vi "Get Disable.vi"(8 "error in (no error)":errorcluster, 11 "S4ACS_GUI in":refnum<class "S4GUI.lvclass">) -> (0 "error out":errorcluster, 3 "S4ACS_GUI out":refnum<class "S4GUI.lvclass">)   [LabVIEW 2018, in "S4GUI.lvclass"]
uses:
  S4GUI.lvclass
  S4GUI.lvclass/S4GUI.ctl
  Server/Server.lvclass/Server.ctl
  Acquisition/Acquisition.lvclass
  C:/Users/devstaff/sparc4/s4gui/Versao ZeroMQ REQ-REP/SPARC4_GUI -v1.0.9 - novo comportamento aba TEST/Server/Server.lvclass
  Instrument/Instrument.lvclass
  Server/Server.lvclass
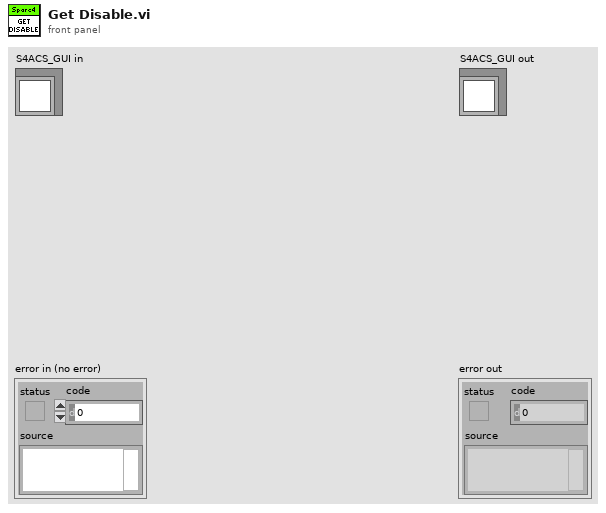
[diagram p1: front panel]
types:
  T1 = enum8{"Enabled", "Disabled", "Disabled and Grayed Out"}
  T2 = cluster{"Cluster Mode Sync":cluster{"#Index Cycles":enum8{"Enabled", "Disabled", "Disabled and Grayed Out"}, "#Cycles":enum8{"Enabled", "Disabled", "Disabled and Grayed Out"}, "SSM":enum8{"Enabled", "Disabled", "Disabled and Grayed Out"}, "Set SM":enum8{"Enabled", "Disabled", "Disabled and Grayed Out"}, "Star SM":enum8{"Enabled", "Disabled", "Disabled and Grayed Out"}, "Pause SM":enum8{"Enabled", "Disabled", "Disabled and Grayed Out"}, "Stop SM":enum8{"Enabled", "Disabled", "Disabled and Grayed Out"}, "Abort SM":enum8{"Enabled", "Disabled", "Disabled and Grayed Out"}, "Start SM Text":string}, "Cluster Polarimetry":cluster{"Lambda Selector":enum8{"Enabled", "Disabled", "Disabled and Grayed Out"}, "Calibrator Selector":enum8{"Enabled", "Disabled", "Disabled and Grayed Out"}, "Set Waveplate":enum8{"Enabled", "Disabled", "Disabled and Grayed Out"}, "Select Positions":enum8{"Enabled", "Disabled", "Disabled and Grayed Out"}, "P0":enum8{"Enabled", "Disabled", "Disabled and Grayed Out"}, "P1":enum8{"Enabled", "Disabled", "Disabled and Grayed Out"}, "P2":enum8{"Enabled", "Disabled", "Disabled and Grayed Out"}, "P3":enum8{"Enabled", "Disabled", "Disabled and Grayed Out"}, "P4":enum8{"Enabled", "Disabled", "Disabled and Grayed Out"}, "P5":enum8{"Enabled", "Disabled", "Disabled and Grayed Out"}, "P6":enum8{"Enabled", "Disabled", "Disabled and Grayed Out"}, "P7":enum8{"Enabled", "Disabled", "Disabled and Grayed Out"}, "P8":enum8{"Enabled", "Disabled", "Disabled and Grayed Out"}, "P9":enum8{"Enabled", "Disabled", "Disabled and Grayed Out"}, "P10":enum8{"Enabled", "Disabled", "Disabled and Grayed Out"}, "P11":enum8{"Enabled", "Disabled", "Disabled and Grayed Out"}, "P12":enum8{"Enabled", "Disabled", "Disabled and Grayed Out"}, "P13":enum8{"Enabled", "Disabled", "Disabled and Grayed Out"}, "P14":enum8{"Enabled", "Disabled", "Disabled and Grayed Out"}, "P15":enum8{"Enabled", "Disabled", "Disabled and Grayed Out"}}, "Cluster Mode CH1":cluster{"#cycles ch1":enum8{"Enabled", "Disabled", "Disabled and Grayed Out"}, "Start ch1":enum8{"Enabled", "Disabled", "Disabled and Grayed Out"}, "Pause ch1":enum8{"Enabled", "Disabled", "Disabled and Grayed Out"}, "Stop ch1":enum8{"Enabled", "Disabled", "Disabled and Grayed Out"}, "Abort ch1":enum8{"Enabled", "Disabled", "Disabled and Grayed Out"}, "Exptime ch1":enum8{"Enabled", "Disabled", "Disabled and Grayed Out"}, "Exp ch1":enum8{"Enabled", "Disabled", "Disabled and Grayed Out"}, "Start ch1 Text":string, "Set Cooler":enum8{"Enabled", "Disabled", "Disabled and Grayed Out"}, "Set Temp":enum8{"Enabled", "Disabled", "Disabled and Grayed Out"}}, "Cluster Mode CH2":cluster{"#cycles ch2":enum8{"Enabled", "Disabled", "Disabled and Grayed Out"}, "Start ch2":enum8{"Enabled", "Disabled", "Disabled and Grayed Out"}, "Pause ch2":enum8{"Enabled", "Disabled", "Disabled and Grayed Out"}, "Stop ch2":enum8{"Enabled", "Disabled", "Disabled and Grayed Out"}, "Abort ch2":enum8{"Enabled", "Disabled", "Disabled and Grayed Out"}, "Exptime ch2":enum8{"Enabled", "Disabled", "Disabled and Grayed Out"}, "Exp ch2":enum8{"Enabled", "Disabled", "Disabled and Grayed Out"}, "Start ch2 Text":string, "Set Cooler":enum8{"Enabled", "Disabled", "Disabled and Grayed Out"}, "Set Temp":enum8{"Enabled", "Disabled", "Disabled and Grayed Out"}}, "Cluster Mode CH3":cluster{"#cycles ch3":enum8{"Enabled", "Disabled", "Disabled and Grayed Out"}, "Start ch3":enum8{"Enabled", "Disabled", "Disabled and Grayed Out"}, "Pause ch3":enum8{"Enabled", "Disabled", "Disabled and Grayed Out"}, "Stop ch3":enum8{"Enabled", "Disabled", "Disabled and Grayed Out"}, "Abort ch3":enum8{"Enabled", "Disabled", "Disabled and Grayed Out"}, "Exptime ch3":enum8{"Enabled", "Disabled", "Disabled and Grayed Out"}, "Exp ch3":enum8{"Enabled", "Disabled", "Disabled and Grayed Out"}, "Start ch3 Text":string, "Set Cooler":enum8{"Enabled", "Disabled", "Disabled and Grayed Out"}, "Set Temp":enum8{"Enabled", "Disabled", "Disabled and Grayed Out"}}, "Cluster Mode CH4":cluster{"#cycles ch4":enum8{"Enabled", "Disabled", "Disabled and Grayed Out"}, "Start ch4":enum8{"Enabled", "Disabled", "Disabled and Grayed Out"}, "Pause ch4":enum8{"Enabled", "Disabled", "Disabled and Grayed Out"}, "Stop ch4":enum8{"Enabled", "Disabled", "Disabled and Grayed Out"}, "Abort ch4":enum8{"Enabled", "Disabled", "Disabled and Grayed Out"}, "Exptime ch4":enum8{"Enabled", "Disabled", "Disabled and Grayed Out"}, "Exp ch4":enum8{"Enabled", "Disabled", "Disabled and Grayed Out"}, "Start ch4 Text":string, "Set Cooler":enum8{"Enabled", "Disabled", "Disabled and Grayed Out"}, "Set Temp":enum8{"Enabled", "Disabled", "Disabled and Grayed Out"}}, "Cluster ExpMode":cluster{"tab4":enum8{"Enabled", "Disabled", "Disabled and Grayed Out"}}, "Cluster AdmCCDsetup":cluster{"param":enum8{"Enabled", "Disabled", "Disabled and Grayed Out"}}}
  T3 = enum32{"OBJECT", "TEST", "DFLAT", "SFLAT", "DARK", "ZERO", "FOCUS"}
  T4 = cluster{"#Index Cycles":enum8{"Enabled", "Disabled", "Disabled and Grayed Out"}, "#Cycles":enum8{"Enabled", "Disabled", "Disabled and Grayed Out"}, "SSM":enum8{"Enabled", "Disabled", "Disabled and Grayed Out"}, "Set SM":enum8{"Enabled", "Disabled", "Disabled and Grayed Out"}, "Star SM":enum8{"Enabled", "Disabled", "Disabled and Grayed Out"}, "Pause SM":enum8{"Enabled", "Disabled", "Disabled and Grayed Out"}, "Stop SM":enum8{"Enabled", "Disabled", "Disabled and Grayed Out"}, "Abort SM":enum8{"Enabled", "Disabled", "Disabled and Grayed Out"}, "Start SM Text":string}
  T5 = cluster{"#cycles ch1":enum8{"Enabled", "Disabled", "Disabled and Grayed Out"}, "Start ch1":enum8{"Enabled", "Disabled", "Disabled and Grayed Out"}, "Pause ch1":enum8{"Enabled", "Disabled", "Disabled and Grayed Out"}, "Stop ch1":enum8{"Enabled", "Disabled", "Disabled and Grayed Out"}, "Abort ch1":enum8{"Enabled", "Disabled", "Disabled and Grayed Out"}, "Exptime ch1":enum8{"Enabled", "Disabled", "Disabled and Grayed Out"}, "Exp ch1":enum8{"Enabled", "Disabled", "Disabled and Grayed Out"}, "Start ch1 Text":string, "Set Cooler":enum8{"Enabled", "Disabled", "Disabled and Grayed Out"}, "Set Temp":enum8{"Enabled", "Disabled", "Disabled and Grayed Out"}}
  T6 = cluster{"#cycles ch2":enum8{"Enabled", "Disabled", "Disabled and Grayed Out"}, "Start ch2":enum8{"Enabled", "Disabled", "Disabled and Grayed Out"}, "Pause ch2":enum8{"Enabled", "Disabled", "Disabled and Grayed Out"}, "Stop ch2":enum8{"Enabled", "Disabled", "Disabled and Grayed Out"}, "Abort ch2":enum8{"Enabled", "Disabled", "Disabled and Grayed Out"}, "Exptime ch2":enum8{"Enabled", "Disabled", "Disabled and Grayed Out"}, "Exp ch2":enum8{"Enabled", "Disabled", "Disabled and Grayed Out"}, "Start ch2 Text":string, "Set Cooler":enum8{"Enabled", "Disabled", "Disabled and Grayed Out"}, "Set Temp":enum8{"Enabled", "Disabled", "Disabled and Grayed Out"}}
  T7 = cluster{"#cycles ch3":enum8{"Enabled", "Disabled", "Disabled and Grayed Out"}, "Start ch3":enum8{"Enabled", "Disabled", "Disabled and Grayed Out"}, "Pause ch3":enum8{"Enabled", "Disabled", "Disabled and Grayed Out"}, "Stop ch3":enum8{"Enabled", "Disabled", "Disabled and Grayed Out"}, "Abort ch3":enum8{"Enabled", "Disabled", "Disabled and Grayed Out"}, "Exptime ch3":enum8{"Enabled", "Disabled", "Disabled and Grayed Out"}, "Exp ch3":enum8{"Enabled", "Disabled", "Disabled and Grayed Out"}, "Start ch3 Text":string, "Set Cooler":enum8{"Enabled", "Disabled", "Disabled and Grayed Out"}, "Set Temp":enum8{"Enabled", "Disabled", "Disabled and Grayed Out"}}
  T8 = cluster{"#cycles ch4":enum8{"Enabled", "Disabled", "Disabled and Grayed Out"}, "Start ch4":enum8{"Enabled", "Disabled", "Disabled and Grayed Out"}, "Pause ch4":enum8{"Enabled", "Disabled", "Disabled and Grayed Out"}, "Stop ch4":enum8{"Enabled", "Disabled", "Disabled and Grayed Out"}, "Abort ch4":enum8{"Enabled", "Disabled", "Disabled and Grayed Out"}, "Exptime ch4":enum8{"Enabled", "Disabled", "Disabled and Grayed Out"}, "Exp ch4":enum8{"Enabled", "Disabled", "Disabled and Grayed Out"}, "Start ch4 Text":string, "Set Cooler":enum8{"Enabled", "Disabled", "Disabled and Grayed Out"}, "Set Temp":enum8{"Enabled", "Disabled", "Disabled and Grayed Out"}}
  T9 = cluster{"Lambda Selector":enum8{"Enabled", "Disabled", "Disabled and Grayed Out"}, "Calibrator Selector":enum8{"Enabled", "Disabled", "Disabled and Grayed Out"}, "Set Waveplate":enum8{"Enabled", "Disabled", "Disabled and Grayed Out"}, "Select Positions":enum8{"Enabled", "Disabled", "Disabled and Grayed Out"}, "P0":enum8{"Enabled", "Disabled", "Disabled and Grayed Out"}, "P1":enum8{"Enabled", "Disabled", "Disabled and Grayed Out"}, "P2":enum8{"Enabled", "Disabled", "Disabled and Grayed Out"}, "P3":enum8{"Enabled", "Disabled", "Disabled and Grayed Out"}, "P4":enum8{"Enabled", "Disabled", "Disabled and Grayed Out"}, "P5":enum8{"Enabled", "Disabled", "Disabled and Grayed Out"}, "P6":enum8{"Enabled", "Disabled", "Disabled and Grayed Out"}, "P7":enum8{"Enabled", "Disabled", "Disabled and Grayed Out"}, "P8":enum8{"Enabled", "Disabled", "Disabled and Grayed Out"}, "P9":enum8{"Enabled", "Disabled", "Disabled and Grayed Out"}, "P10":enum8{"Enabled", "Disabled", "Disabled and Grayed Out"}, "P11":enum8{"Enabled", "Disabled", "Disabled and Grayed Out"}, "P12":enum8{"Enabled", "Disabled", "Disabled and Grayed Out"}, "P13":enum8{"Enabled", "Disabled", "Disabled and Grayed Out"}, "P14":enum8{"Enabled", "Disabled", "Disabled and Grayed Out"}, "P15":enum8{"Enabled", "Disabled", "Disabled and Grayed Out"}}
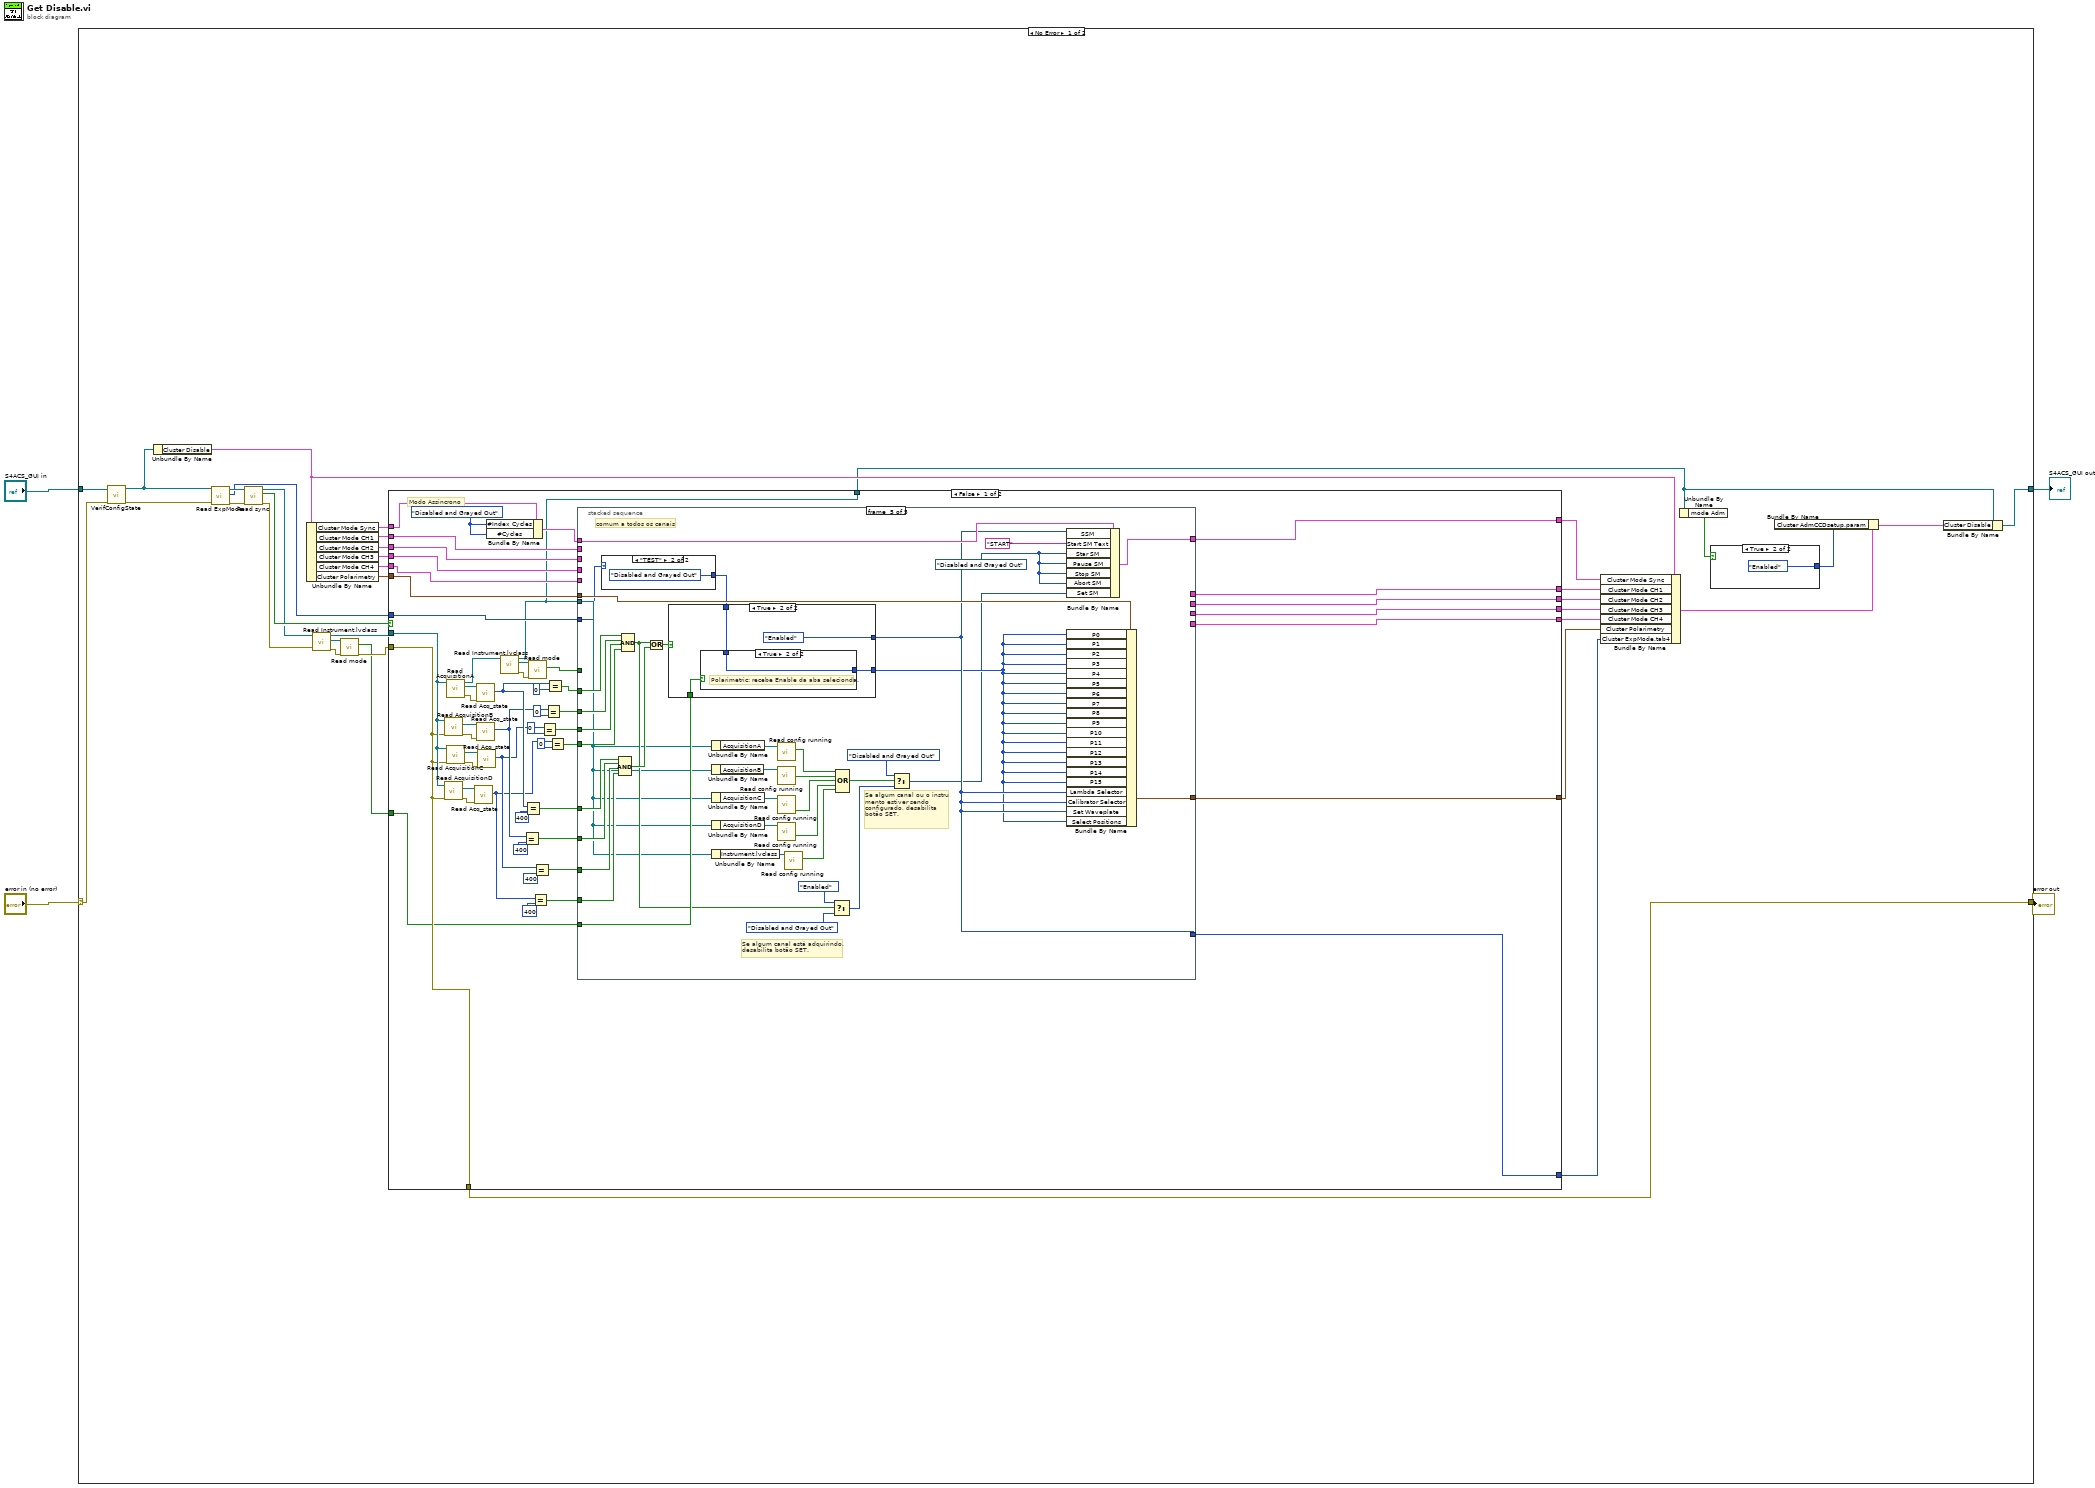
[diagram p0: block diagram]
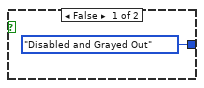
[diagram p2: hidden frame]
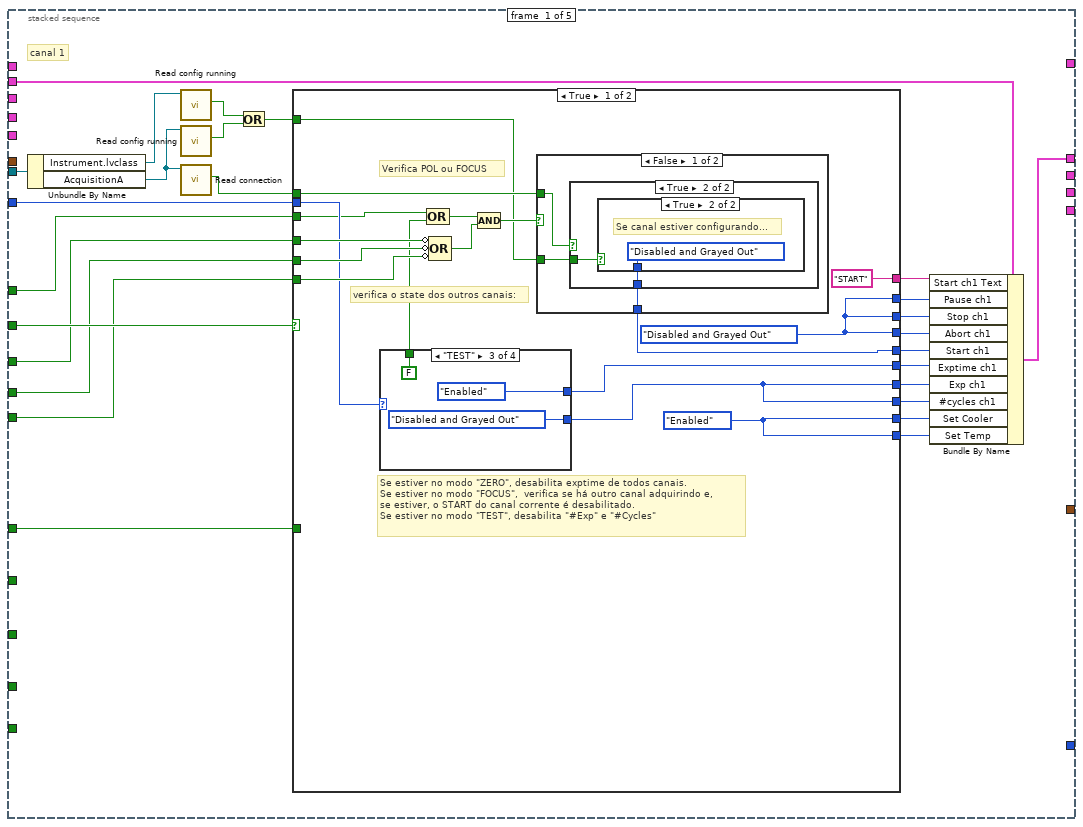
[diagram p3: hidden frame]
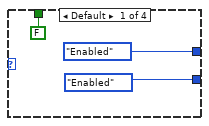
[diagram p4: hidden frame]
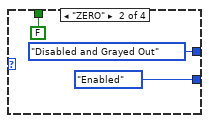
[diagram p5: hidden frame]
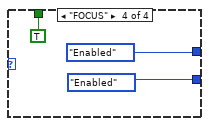
[diagram p6: hidden frame]
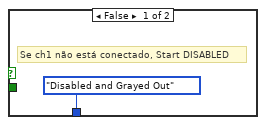
[diagram p7: hidden frame]
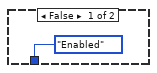
[diagram p8: hidden frame]
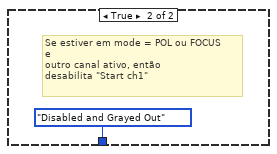
[diagram p9: hidden frame]
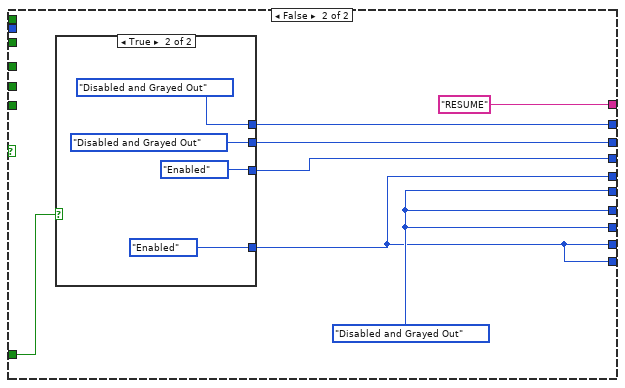
[diagram p10: hidden frame]
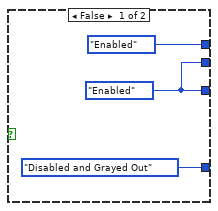
[diagram p11: hidden frame]
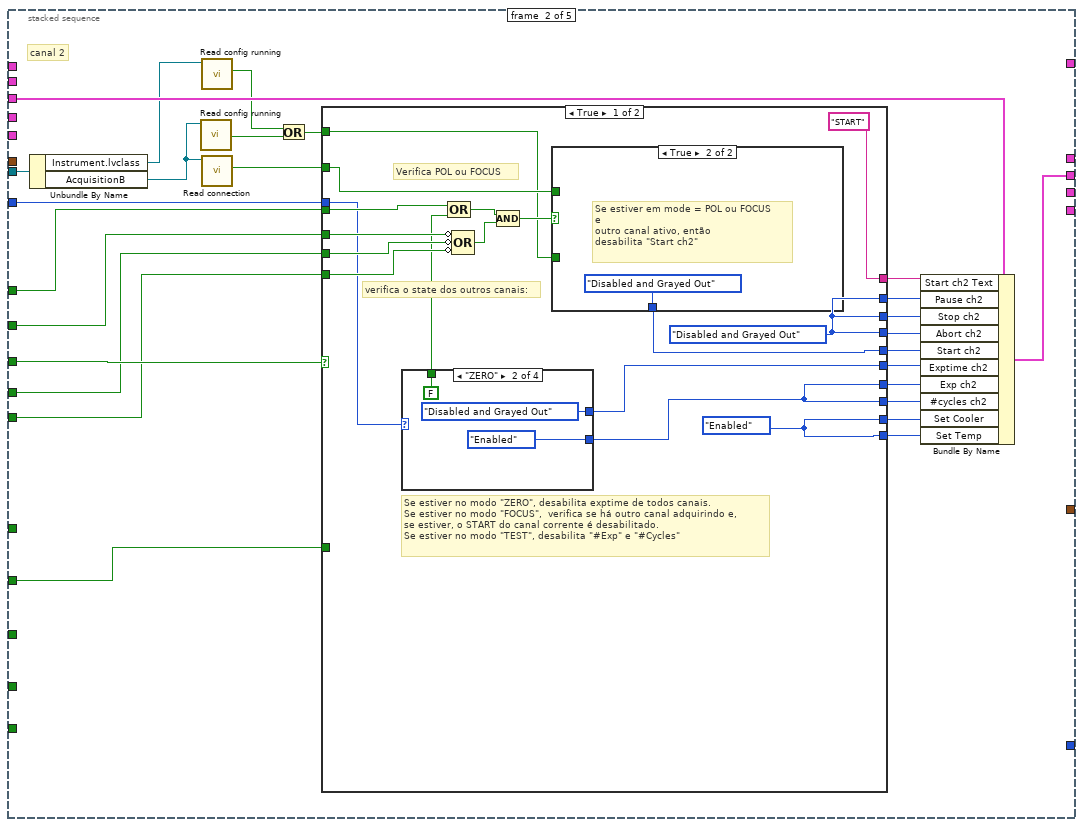
[diagram p12: hidden frame]
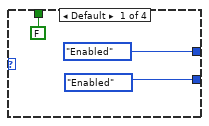
[diagram p13: hidden frame]
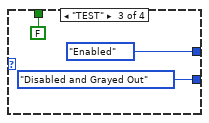
[diagram p14: hidden frame]
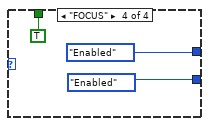
[diagram p15: hidden frame]
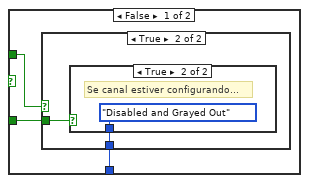
[diagram p16: hidden frame]
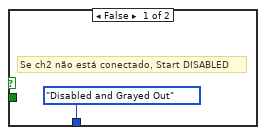
[diagram p17: hidden frame]
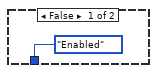
[diagram p18: hidden frame]
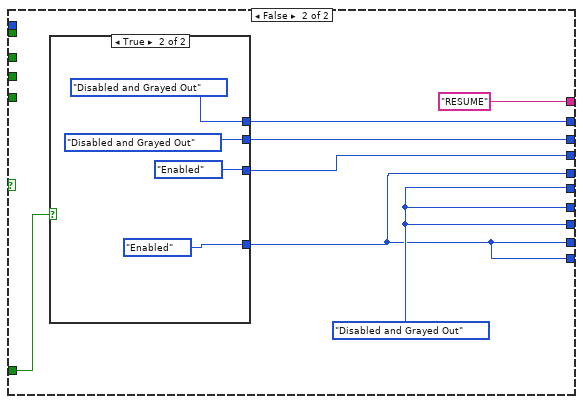
[diagram p19: hidden frame]
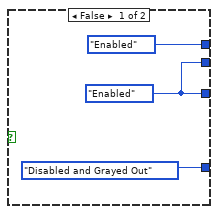
[diagram p20: hidden frame]
diagram:
  n1 = case shown="No Error" "error in (no error)" {
    selector: "error in (no error)" -> [w21 w567]
    tunnel: [w33 w567] -> w3
    tunnel: [w5 w566] -> w1
    tunnel: "S4ACS_GUI in" -> [w22 w566]
    frame No Error {
      n2 = call-dynamic "VerifConfigState.vi"("error in (no error)"=w21, "S4GUI in"=w22) -> ("error out"=w9:errorcluster, "S4GUI out"=w8:refnum<class "S4GUI.lvclass">)  [unwired: 8 in]
      n3 = Unbundle By Name(w8) -> ("Cluster Disable"=w7:T2)
      n4 = call-dynamic "Read ExpMode.vi"("error in (no error)"=w9, "S4GUI in"=w8) -> ("error out"=w24:errorcluster, "ExpMode"=w23:T3, "S4GUI out"=w25:refnum<class "S4GUI.lvclass">)  [unwired: 7 in]
      n5 = call-dynamic "Read sync.vi"("error in (no error)"=w24, "S4ACS_GUI in"=w25) -> ("error out"=w14:errorcluster, "sync"=w40:bool, "S4ACS_GUI out"=w16:refnum<class "S4GUI.lvclass">)  [unwired: 7 in]
      n6 = Unbundle By Name(w7) -> ("Cluster Mode Sync"=w39:T4, "Cluster Mode CH1"=w38:T5, "Cluster Mode CH2"=w37:T6, "Cluster Mode CH3"=w31:T7, "Cluster Mode CH4"=w30:T8, "Cluster Polarimetry"=w32:T9)
      n7 = call "Read Instrument.lvclass.vi"("error in (no error)"=w14, "S4ACS_GUI in"=w16) -> ("error out"=w13:errorcluster, "Instrument.lvclass"=w17:refnum<class "Instrument.lvclass">, "S4ACS_GUI out"=w15:refnum<class "S4GUI.lvclass">)  [unwired: 7 in]
      n8 = call-dynamic "Read mode.vi"("error in (no error)"=w13, "Instrument in"=w17) -> ("error out"=w12:errorcluster, "mode"=w11:bool)  [unwired: 7 in, 1 out]
      n9 = case shown="False" w40 {
        tunnel: w15 -> [w63 w492]
        tunnel: w12 -> [w62 w491]
        tunnel: w39 -> [w76 w490]
        tunnel: w38 -> [w74 w482]
        tunnel: w37 -> [w72 w479]
        tunnel: [w73 w488] -> w36
        tunnel: [w51 w480] -> w35
        tunnel: w32 -> [w71 w487]
        tunnel: [w70 w478] -> w29
        tunnel: [w50 w481] -> w34
        tunnel: [w62 w477] -> w33
        tunnel: [w46 w461] -> w6
        tunnel: w31 -> [w69 w473]
        tunnel: w30 -> [w68 w469]
        tunnel: [w49 w472] -> w28
        tunnel: [w48 w468] -> w27
        tunnel: [w45 w467] -> w26
        tunnel: w23 -> [w47 w466]
        tunnel: w11 -> [w43 w456]
        frame False {
          w44 = T1."Disabled and Grayed Out" ("Disabled")
          # "Modo Assincrono"
          n10 = call-dynamic "Read AcquisitionD.vi"("error in (no error)"=w62, "S4ACS_GUI in"=w63) -> ("error out"=w64:errorcluster, "Acquisition.lvclass"=w65:refnum<class "Acquisition.lvclass">)  [unwired: 7 in, 1 out]
          n11 = call "Read AcquisitionB.vi"("error in (no error)"=w62, "S4ACS_GUI in"=w63) -> ("error out"=w91:errorcluster, "Acquisition.lvclass"=w92:refnum<class "Acquisition.lvclass">)  [unwired: 7 in, 1 out]
          n12 = call-dynamic "Read AcquisitionC.vi"("error in (no error)"=w62, "S4ACS_GUI in"=w63) -> ("error out"=w67:errorcluster, "Acquisition.lvclass"=w66:refnum<class "Acquisition.lvclass">)  [unwired: 7 in, 1 out]
          n13 = call-dynamic "Read AcquisitionA.vi"("S4ACS_GUI in"=w63) -> ("error out"=w93:errorcluster, "Acquisition.lvclass"=w94:refnum<class "Acquisition.lvclass">, "S4ACS_GUI out"=w77:refnum<class "S4GUI.lvclass">)  [unwired: 8 in]
          n14 = call-dynamic "Read Acq_state.vi"("error in (no error)"=w64, "Acquisition in"=w65) -> ("Acq_state"=w54:u32)  [unwired: 7 in, 2 out]
          n15 = call-dynamic "Read Acq_state.vi"("error in (no error)"=w93, "Acquisition in"=w94) -> ("Acq_state"=w84:u32)  [unwired: 7 in, 2 out]
          n16 = call-dynamic "Read Acq_state.vi"("error in (no error)"=w91, "Acquisition in"=w92) -> ("Acq_state"=w81:u32)  [unwired: 7 in, 2 out]
          n17 = call-dynamic "Read Acq_state.vi"("error in (no error)"=w67, "Acquisition in"=w66) -> ("Acq_state"=w55:u32)  [unwired: 7 in, 2 out]
          n18 = Bundle By Name(cluster=w76, "#Index Cycles"=w44, "#Cycles"=w44) -> (w75:T4)
          n19 = call "Read Instrument.lvclass.vi"("S4ACS_GUI in"=w77) -> ("error out"=w79:errorcluster, "Instrument.lvclass"=w80:refnum<class "Instrument.lvclass">, "S4ACS_GUI out"=w46:refnum<class "S4GUI.lvclass">)  [unwired: 8 in]
          n20 = Equal?(x=w81, y=u32 400) -> (x = y?=w85:bool)
          n21 = Equal?(x=w84, y=u32 400) -> (x = y?=w86:bool)
          n22 = call-dynamic "Read mode.vi"("error in (no error)"=w79, "Instrument in"=w80) -> ("mode"=w78:bool)  [unwired: 7 in, 2 out]
          n23 = Equal?(x=w54, y=u32 400) -> (x = y?=w52:bool)
          n24 = Equal?(x=w55, y=u32 400) -> (x = y?=w53:bool)
          n25 = Equal?(x=w55, y=u32 0) -> (x = y?=w59:bool)
          n26 = Equal?(x=w81, y=u32 0) -> (x = y?=w83:bool)
          n27 = Equal?(x=w84, y=u32 0) -> (x = y?=w89:bool)
          n28 = Equal?(x=w54, y=u32 0) -> (x = y?=w60:bool)
          n29 = stacked-sequence {
            tunnel: w89 -> [w120 w187 w267 w345 w445]
            tunnel: w86 -> [w119 _ _ _ w443]
            tunnel: w85 -> [_ w185 _ _ w442]
            tunnel: w83 -> [w117 w186 w264 w341 w444]
            tunnel: w78 -> [w118 w198 w276 w354 _]
            tunnel: w75 -> [_ _ _ _ w437]
            tunnel: w74 -> [w116 _ _ _ _]
            tunnel: [_ _ _ _ w436] -> w73
            tunnel: [w107 _ _ _ _] -> w51
            tunnel: w72 -> [_ w189 _ _ _]
            tunnel: w71 -> [_ _ _ _ w439]
            tunnel: [_ _ _ _ w438] -> w70
            tunnel: [_ w188 _ _ _] -> w50
            tunnel: w69 -> [_ _ w266 _ _]
            tunnel: w68 -> [_ _ _ w344 _]
            tunnel: [_ _ w265 _ _] -> w49
            tunnel: [_ _ _ w343 _] -> w48
            tunnel: w59 -> [w106 w184 w263 w340 w433]
            tunnel: w60 -> [w105 w183 w262 w342 w432]
            tunnel: w53 -> [_ _ w261 _ w431]
            tunnel: w52 -> [_ _ _ w339 w430]
            tunnel: w47 -> [w104 w182 w260 w338 w408]
            tunnel: w46 -> [w101 w178 w256 w335 w410]
            tunnel: [_ _ _ _ w429] -> w45
            tunnel: w43 -> [_ _ _ _ w427]
            frame #0 {
              # "canal 1"
              n30 = Unbundle By Name(w101) -> ("Instrument.lvclass"=w95:refnum<class "Instrument.lvclass">, "AcquisitionA"=w99:refnum<class "Acquisition.lvclass">)
              n31 = call-dynamic "Read config running.vi"("Server in"=w95) -> ("config running"=w96:bool)  [unwired: 8 in, 2 out]
              n32 = call-dynamic "Read config running.vi"("Server in"=w99) -> ("config running"=w97:bool)  [unwired: 8 in, 2 out]
              n33 = call "Read connection.vi"("Server in"=w99) -> ("connection"=w100:bool)  [unwired: 8 in, 2 out]
              n34 = Or(x=w96, y=w97) -> (x .or. y?=w98:bool)
              n35 = case shown="True" w120 {
                tunnel: w119 -> [_ w165]
                tunnel: w118 -> [w125 _]
                tunnel: w117 -> [w133 _]
                tunnel: ["START" ("Caption.Text") "RESUME" ("Caption.Text")] -> w115
                tunnel: [w135 w163] -> w114
                tunnel: [w135 w159] -> w113
                tunnel: [w135 w160] -> w112
                tunnel: [w134 w161] -> w111
                tunnel: [w128 w162] -> w110
                tunnel: [w121 w162] -> w109
                tunnel: [w121 w162] -> w108
                tunnel: w106 -> [w132 _]
                tunnel: w105 -> [w131 _]
                tunnel: w104 -> [w129 _]
                tunnel: [w122 w161] -> w103
                tunnel: [w122 w161] -> w102
                tunnel: w100 -> [w127 _]
                tunnel: w98 -> [w126 _]
                frame True {
                  w135 = T1."Disabled and Grayed Out" ("Disabled")
                  w122 = T1."Enabled" ("Disabled")
                  # "Verifica POL ou FOCUS"
                  # "Se estiver no modo \"ZERO\", desabilita exptime de todos canais.\nSe estiver no modo \"FOCUS\",  verifica se há outro canal adquirindo e,\nse estiver, o START do canal corrente é desabilitado.\nSe estiver no modo \"TEST\", desabilita \"#Exp\" e \"#Cycles\""
                  # "verifica o state dos outros canais:"
                  n36 = case shown="\"TEST\"" w129 {
                    tunnel: [T1."Enabled" ("Disabled") T1."Disabled and Grayed Out" ("Disabled") T1."Enabled" ("Disabled") T1."Enabled" ("Disabled")] -> w128
                    tunnel: [FALSE FALSE FALSE TRUE] -> w123
                    tunnel: [T1."Enabled" ("Disabled") T1."Enabled" ("Disabled") T1."Disabled and Grayed Out" ("Disabled") T1."Enabled" ("Disabled")] -> w121
                    frame Default {
                    }
                    frame "ZERO" {
                    }
                    frame "TEST" {
                    }
                    frame "FOCUS" {
                    }
                  }
                  n37 = Compound Arithmetic op=OR(w125, w123) -> (w124:bool)
                  n38 = Compound Arithmetic op=OR(invert w133, invert w132, invert w131) -> (w130:bool)
                  n39 = Compound Arithmetic op=AND(w124, w130) -> (w137:bool)
                  n40 = case shown="False" w137 {
                    tunnel: [w152 T1."Disabled and Grayed Out" ("Disabled")] -> w134
                    tunnel: w127 -> [w151 _]
                    tunnel: w126 -> [w150 _]
                    frame False {
                      n41 = case shown="True" w151 {
                        tunnel: [T1."Disabled and Grayed Out" ("Disabled") w155] -> w152
                        tunnel: w150 -> [_ w154]
                        frame False {
                          # "Se ch1 não está conectado, Start DISABLED"
                        }
                        frame True {
                          n42 = case shown="True" w154 {
                            tunnel: [T1."Enabled" ("Disabled") T1."Disabled and Grayed Out" ("Disabled")] -> w155
                            frame False {
                            }
                            frame True {
                              # "Se canal estiver configurando..."
                            }
                          }
                        }
                      }
                    }
                    frame True {
                      # "Se estiver em mode = POL ou FOCUS\ne\noutro canal ativo, então\ndesabilita \"Start ch1\""
                    }
                  }
                }
                frame False {
                  w162 = T1."Disabled and Grayed Out" ("Disabled")
                  n43 = case shown="True" w165 {
                    tunnel: [T1."Enabled" ("Disabled") T1."Disabled and Grayed Out" ("Disabled")] -> w163
                    tunnel: [T1."Disabled and Grayed Out" ("Disabled") T1."Enabled" ("Disabled")] -> w161
                    tunnel: [w166 T1."Enabled" ("Disabled")] -> w160
                    tunnel: [w166 T1."Disabled and Grayed Out" ("Disabled")] -> w159
                    frame False {
                      w166 = T1."Enabled" ("Disabled")
                    }
                    frame True {
                    }
                  }
                }
              }
              n44 = Bundle By Name(cluster=w116, "Start ch1 Text"=w115, "Pause ch1"=w114, "Stop ch1"=w113, "Abort ch1"=w112, "Start ch1"=w111, "Exptime ch1"=w110, "Exp ch1"=w109, "#cycles ch1"=w108, "Set Cooler"=w103, "Set Temp"=w102) -> (w107:T5)
            }
            frame #1 {
              # "canal 2"
              n45 = Unbundle By Name(w178) -> ("Instrument.lvclass"=w173:refnum<class "Instrument.lvclass">, "AcquisitionB"=w179:refnum<class "Acquisition.lvclass">)
              n46 = call-dynamic "Read config running.vi"("Server in"=w179) -> ("config running"=w174:bool)  [unwired: 8 in, 2 out]
              n47 = call-dynamic "Read config running.vi"("Server in"=w173) -> ("config running"=w175:bool)  [unwired: 8 in, 2 out]
              n48 = call "Read connection.vi"("Server in"=w179) -> ("connection"=w177:bool)  [unwired: 8 in, 2 out]
              n49 = Or(x=w175, y=w174) -> (x .or. y?=w176:bool)
              n50 = case shown="True" w186 {
                tunnel: w185 -> [_ w241]
                tunnel: w198 -> [w204 _]
                tunnel: w187 -> [w212 _]
                tunnel: ["START" ("Caption.Text") "RESUME" ("Caption.Text")] -> w197
                tunnel: [w214 w239] -> w196
                tunnel: [w214 w238] -> w195
                tunnel: [w214 w237] -> w194
                tunnel: [w206 w240] -> w193
                tunnel: [w200 w242] -> w192
                tunnel: [w199 w242] -> w191
                tunnel: [w199 w242] -> w190
                tunnel: w184 -> [w211 _]
                tunnel: w183 -> [w210 _]
                tunnel: w182 -> [w201 _]
                tunnel: [w203 w240] -> w181
                tunnel: [w203 w240] -> w180
                tunnel: w177 -> [w208 _]
                tunnel: w176 -> [w207 _]
                frame True {
                  w214 = T1."Disabled and Grayed Out" ("Disabled")
                  w203 = T1."Enabled" ("Disabled")
                  # "Se estiver no modo \"ZERO\", desabilita exptime de todos canais.\nSe estiver no modo \"FOCUS\",  verifica se há outro canal adquirindo e,\nse estiver, o START do canal corrente é desabilitado.\nSe estiver no modo \"TEST\", desabilita \"#Exp\" e \"#Cycles\""
                  # "Verifica POL ou FOCUS"
                  # "verifica o state dos outros canais:"
                  n51 = case shown="\"ZERO\"" w201 {
                    tunnel: [T1."Enabled" ("Disabled") T1."Disabled and Grayed Out" ("Disabled") T1."Enabled" ("Disabled") T1."Enabled" ("Disabled")] -> w200
                    tunnel: [FALSE FALSE FALSE TRUE] -> w202
                    tunnel: [T1."Enabled" ("Disabled") T1."Enabled" ("Disabled") T1."Disabled and Grayed Out" ("Disabled") T1."Enabled" ("Disabled")] -> w199
                    frame Default {
                    }
                    frame "ZERO" {
                    }
                    frame "TEST" {
                    }
                    frame "FOCUS" {
                    }
                  }
                  n52 = Compound Arithmetic op=OR(w204, w202) -> (w205:bool)
                  n53 = Compound Arithmetic op=OR(invert w212, invert w211, invert w210) -> (w213:bool)
                  n54 = Compound Arithmetic op=AND(w205, w213) -> (w209:bool)
                  n55 = case shown="True" w209 {
                    tunnel: [w230 T1."Disabled and Grayed Out" ("Disabled")] -> w206
                    tunnel: w208 -> [w229 _]
                    tunnel: w207 -> [w228 _]
                    frame False {
                      n56 = case shown="True" w229 {
                        tunnel: [T1."Disabled and Grayed Out" ("Disabled") w233] -> w230
                        tunnel: w228 -> [_ w232]
                        frame False {
                          # "Se ch2 não está conectado, Start DISABLED"
                        }
                        frame True {
                          n57 = case shown="True" w232 {
                            tunnel: [T1."Enabled" ("Disabled") T1."Disabled and Grayed Out" ("Disabled")] -> w233
                            frame False {
                            }
                            frame True {
                              # "Se canal estiver configurando..."
                            }
                          }
                        }
                      }
                    }
                    frame True {
                      # "Se estiver em mode = POL ou FOCUS\ne\noutro canal ativo, então\ndesabilita \"Start ch2\""
                    }
                  }
                }
                frame False {
                  w242 = T1."Disabled and Grayed Out" ("Disabled")
                  n58 = case shown="True" w241 {
                    tunnel: [T1."Enabled" ("Disabled") T1."Disabled and Grayed Out" ("Disabled")] -> w239
                    tunnel: [T1."Disabled and Grayed Out" ("Disabled") T1."Enabled" ("Disabled")] -> w240
                    tunnel: [w244 T1."Enabled" ("Disabled")] -> w237
                    tunnel: [w244 T1."Disabled and Grayed Out" ("Disabled")] -> w238
                    frame False {
                      w244 = T1."Enabled" ("Disabled")
                    }
                    frame True {
                    }
                  }
                }
              }
              n59 = Bundle By Name(cluster=w189, "Start ch2 Text"=w197, "Pause ch2"=w196, "Stop ch2"=w195, "Abort ch2"=w194, "Start ch2"=w193, "Exptime ch2"=w192, "Exp ch2"=w191, "#cycles ch2"=w190, "Set Cooler"=w181, "Set Temp"=w180) -> (w188:T6)
            }
            frame #2 {
              # "canal 3"
              n60 = Unbundle By Name(w256) -> ("Instrument.lvclass"=w253:refnum<class "Instrument.lvclass">, "AcquisitionC"=w257:refnum<class "Acquisition.lvclass">)
              n61 = call-dynamic "Read config running.vi"("Server in"=w253) -> ("config running"=w252:bool)  [unwired: 8 in, 2 out]
              n62 = call-dynamic "Read config running.vi"("Server in"=w257) -> ("config running"=w251:bool)  [unwired: 8 in, 2 out]
              n63 = call "Read connection.vi"("Server in"=w257) -> ("connection"=w255:bool)  [unwired: 8 in, 2 out]
              n64 = Or(x=w252, y=w251) -> (x .or. y?=w254:bool)
              n65 = case shown="True" w263 {
                tunnel: w261 -> [_ w319]
                tunnel: w276 -> [w282 _]
                tunnel: w267 -> [w290 _]
                tunnel: ["START" ("Caption.Text") "RESUME" ("Caption.Text")] -> w275
                tunnel: [w292 w318] -> w274
                tunnel: [w292 w316] -> w273
                tunnel: [w292 w315] -> w272
                tunnel: [w287 w317] -> w271
                tunnel: [w278 w320] -> w270
                tunnel: [w277 w320] -> w269
                tunnel: [w277 w320] -> w268
                tunnel: w264 -> [w289 _]
                tunnel: w262 -> [w288 _]
                tunnel: w260 -> [w279 _]
                tunnel: [w281 w317] -> w259
                tunnel: [w281 w317] -> w258
                tunnel: w255 -> [w285 _]
                tunnel: w254 -> [w284 _]
                frame True {
                  w292 = T1."Disabled and Grayed Out" ("Disabled")
                  w281 = T1."Enabled" ("Disabled")
                  # "Se estiver no modo \"ZERO\", desabilita exptime de todos canais.\nSe estiver no modo \"FOCUS\",  verifica se há outro canal adquirindo e,\nse estiver, o START do canal corrente é desabilitado.\nSe estiver no modo \"TEST\", desabilita \"#Exp\" e \"#Cycles\""
                  # "Verifica POL ou FOCUS"
                  # "verifica o state dos outros canais:"
                  n66 = case shown="\"TEST\"" w279 {
                    tunnel: [T1."Enabled" ("Disabled") T1."Disabled and Grayed Out" ("Disabled") T1."Enabled" ("Disabled") T1."Enabled" ("Disabled")] -> w278
                    tunnel: [FALSE FALSE FALSE TRUE] -> w280
                    tunnel: [T1."Enabled" ("Disabled") T1."Enabled" ("Disabled") T1."Disabled and Grayed Out" ("Disabled") T1."Enabled" ("Disabled")] -> w277
                    frame Default {
                    }
                    frame "ZERO" {
                    }
                    frame "TEST" {
                    }
                    frame "FOCUS" {
                    }
                  }
                  n67 = Compound Arithmetic op=OR(w282, w280) -> (w283:bool)
                  n68 = Compound Arithmetic op=OR(invert w290, invert w289, invert w288) -> (w291:bool)
                  n69 = Compound Arithmetic op=AND(w283, w291) -> (w286:bool)
                  n70 = case shown="True" w286 {
                    tunnel: [w308 T1."Disabled and Grayed Out" ("Disabled")] -> w287
                    tunnel: w285 -> [w307 _]
                    tunnel: w284 -> [w306 _]
                    frame False {
                      n71 = case shown="True" w307 {
                        tunnel: [T1."Disabled and Grayed Out" ("Disabled") w311] -> w308
                        tunnel: w306 -> [_ w310]
                        frame False {
                          # "Se ch3 não está conectado, Start DISABLED"
                        }
                        frame True {
                          n72 = case shown="True" w310 {
                            tunnel: [T1."Enabled" ("Disabled") T1."Disabled and Grayed Out" ("Disabled")] -> w311
                            frame False {
                            }
                            frame True {
                              # "Se canal estiver configurando..."
                            }
                          }
                        }
                      }
                    }
                    frame True {
                      # "Se estiver em mode = POL ou FOCUS\ne\noutro canal ativo, então\ndesabilita \"Start ch3\""
                    }
                  }
                }
                frame False {
                  w320 = T1."Disabled and Grayed Out" ("Disabled")
                  n73 = case shown="True" w319 {
                    tunnel: [T1."Enabled" ("Disabled") T1."Disabled and Grayed Out" ("Disabled")] -> w318
                    tunnel: [T1."Disabled and Grayed Out" ("Disabled") T1."Enabled" ("Disabled")] -> w317
                    tunnel: [w322 T1."Enabled" ("Disabled")] -> w315
                    tunnel: [w322 T1."Disabled and Grayed Out" ("Disabled")] -> w316
                    frame False {
                      w322 = T1."Enabled" ("Disabled")
                    }
                    frame True {
                    }
                  }
                }
              }
              n74 = Bundle By Name(cluster=w266, "Start ch3 Text"=w275, "Pause ch3"=w274, "Stop ch3"=w273, "Abort ch3"=w272, "Start ch3"=w271, "Exptime ch3"=w270, "Exp ch3"=w269, "#cycles ch3"=w268, "Set Cooler"=w259, "Set Temp"=w258) -> (w265:T7)
            }
            frame #3 {
              # "canal 4"
              n75 = Unbundle By Name(w335) -> ("Instrument.lvclass"=w331:refnum<class "Instrument.lvclass">, "AcquisitionD"=w334:refnum<class "Acquisition.lvclass">)
              n76 = call-dynamic "Read config running.vi"("Server in"=w331) -> ("config running"=w330:bool)  [unwired: 8 in, 2 out]
              n77 = call-dynamic "Read config running.vi"("Server in"=w334) -> ("config running"=w329:bool)  [unwired: 8 in, 2 out]
              n78 = call "Read connection.vi"("Server in"=w334) -> ("connection"=w333:bool)  [unwired: 8 in, 2 out]
              n79 = Or(x=w330, y=w329) -> (x .or. y?=w332:bool)
              n80 = case shown="True" w342 {
                tunnel: w339 -> [_ w395]
                tunnel: w354 -> [w360 _]
                tunnel: w345 -> [w368 _]
                tunnel: ["START" ("Caption.Text") "RESUME" ("Caption.Text")] -> w353
                tunnel: [w370 w397] -> w352
                tunnel: [w370 w394] -> w351
                tunnel: [w370 w393] -> w350
                tunnel: [w365 w396] -> w349
                tunnel: [w356 w398] -> w348
                tunnel: [w355 w398] -> w347
                tunnel: [w355 w398] -> w346
                tunnel: w341 -> [w367 _]
                tunnel: w340 -> [w366 _]
                tunnel: w338 -> [w357 _]
                tunnel: [w359 w396] -> w337
                tunnel: [w359 w396] -> w336
                tunnel: w332 -> [w362 _]
                tunnel: w333 -> [w363 _]
                frame True {
                  w370 = T1."Disabled and Grayed Out" ("Disabled")
                  w359 = T1."Enabled" ("Disabled")
                  # "Se estiver no modo \"ZERO\", desabilita exptime de todos canais.\nSe estiver no modo \"FOCUS\",  verifica se há outro canal adquirindo e,\nse estiver, o START do canal corrente é desabilitado.\nSe estiver no modo \"TEST\", desabilita \"#Exp\" e \"#Cycles\""
                  # "Verifica POL ou FOCUS"
                  # "verifica o state dos outros canais:"
                  n81 = case shown="\"TEST\"" w357 {
                    tunnel: [T1."Enabled" ("Disabled") T1."Disabled and Grayed Out" ("Disabled") T1."Enabled" ("Disabled") T1."Enabled" ("Disabled")] -> w356
                    tunnel: [FALSE FALSE FALSE TRUE] -> w358
                    tunnel: [T1."Enabled" ("Disabled") T1."Enabled" ("Disabled") T1."Disabled and Grayed Out" ("Disabled") T1."Enabled" ("Disabled")] -> w355
                    frame Default {
                    }
                    frame "ZERO" {
                    }
                    frame "TEST" {
                    }
                    frame "FOCUS" {
                    }
                  }
                  n82 = Compound Arithmetic op=OR(invert w368, invert w367, invert w366) -> (w369:bool)
                  n83 = Compound Arithmetic op=OR(w360, w358) -> (w361:bool)
                  n84 = Compound Arithmetic op=AND(w361, w369) -> (w364:bool)
                  n85 = case shown="False" w364 {
                    tunnel: [w386 T1."Disabled and Grayed Out" ("Disabled")] -> w365
                    tunnel: w363 -> [w385 _]
                    tunnel: w362 -> [w384 _]
                    frame False {
                      n86 = case shown="True" w385 {
                        tunnel: [T1."Disabled and Grayed Out" ("Disabled") w389] -> w386
                        tunnel: w384 -> [_ w388]
                        frame False {
                          # "Se ch4 não está conectado, Start DISABLED"
                        }
                        frame True {
                          n87 = case shown="False" w388 {
                            tunnel: [T1."Enabled" ("Disabled") T1."Disabled and Grayed Out" ("Disabled")] -> w389
                            frame False {
                            }
                            frame True {
                              # "Se canal estiver configurando..."
                            }
                          }
                        }
                      }
                    }
                    frame True {
                      # "Se estiver em mode = POL ou FOCUS\ne\noutro canal ativo, então\ndesabilita \"Start ch4\""
                    }
                  }
                }
                frame False {
                  w398 = T1."Disabled and Grayed Out" ("Disabled")
                  n88 = case shown="True" w395 {
                    tunnel: [T1."Enabled" ("Disabled") T1."Disabled and Grayed Out" ("Disabled")] -> w397
                    tunnel: [T1."Disabled and Grayed Out" ("Disabled") T1."Enabled" ("Disabled")] -> w396
                    tunnel: [w400 T1."Enabled" ("Disabled")] -> w393
                    tunnel: [w400 T1."Disabled and Grayed Out" ("Disabled")] -> w394
                    frame False {
                      w400 = T1."Enabled" ("Disabled")
                    }
                    frame True {
                    }
                  }
                }
              }
              n89 = Bundle By Name(cluster=w344, "Start ch4 Text"=w353, "Pause ch4"=w352, "Stop ch4"=w351, "Abort ch4"=w350, "Start ch4"=w349, "Exptime ch4"=w348, "Exp ch4"=w347, "#cycles ch4"=w346, "Set Cooler"=w337, "Set Temp"=w336) -> (w343:T8)
            }
            frame #4 {
              w434 = T1."Disabled and Grayed Out" ("Disabled")
              # "Se algum canal ou o instru\nmento estiver sendo \nconfigurado, desabilita \nbotão SET."
              # "Se algum canal está adquirindo, \ndesabilita botão SET."
              # "comum a todos os canais"
              n90 = case shown="\"TEST\"" w408 {
                tunnel: [T1."Enabled" ("Disabled") T1."Disabled and Grayed Out" ("Disabled")] -> w407
                frame Default {
                }
                frame "TEST" {
                }
              }
              n91 = Compound Arithmetic op=AND(w443, w442, w431, w430) -> (w440:bool)
              n92 = Compound Arithmetic op=AND(w445, w444, w433, w432) -> (w416:bool)
              n93 = Or(x=w416, y=w440) -> (x .or. y?=w441:bool)
              n94 = case shown="True" w441 {
                tunnel: [w448 T1."Enabled" ("Disabled")] -> w429
                tunnel: [w448 w451] -> w428
                tunnel: w427 -> [_ w450]
                tunnel: w407 -> [_ w449]
                frame False {
                  w448 = T1."Disabled and Grayed Out" ("Disabled")
                }
                frame True {
                  n95 = case shown="True" w450 {
                    tunnel: [T1."Disabled and Grayed Out" ("Disabled") w454] -> w451
                    tunnel: w449 -> [_ w454]
                    frame False {
                      # "Photometric"
                    }
                    frame True {
                      # "Polarimetric: recebe Enable da aba selecionda."
                    }
                  }
                }
              }
              n96 = Unbundle By Name(w410) -> ("Instrument.lvclass"=w411:refnum<class "Instrument.lvclass">)
              n97 = Unbundle By Name(w410) -> ("AcquisitionA"=w422:refnum<class "Acquisition.lvclass">)
              n98 = Unbundle By Name(w410) -> ("AcquisitionB"=w421:refnum<class "Acquisition.lvclass">)
              n99 = Unbundle By Name(w410) -> ("AcquisitionC"=w420:refnum<class "Acquisition.lvclass">)
              n100 = Unbundle By Name(w410) -> ("AcquisitionD"=w419:refnum<class "Acquisition.lvclass">)
              n101 = call-dynamic "Read config running.vi"("Server in"=w422) -> ("config running"=w426:bool)  [unwired: 8 in, 2 out]
              n102 = call-dynamic "Read config running.vi"("Server in"=w421) -> ("config running"=w425:bool)  [unwired: 8 in, 2 out]
              n103 = call-dynamic "Read config running.vi"("Server in"=w420) -> ("config running"=w424:bool)  [unwired: 8 in, 2 out]
              n104 = call-dynamic "Read config running.vi"("Server in"=w419) -> ("config running"=w423:bool)  [unwired: 8 in, 2 out]
              n105 = call-dynamic "Read config running.vi"("Server in"=w411) -> ("config running"=w409:bool)  [unwired: 8 in, 2 out]
              n106 = Select(t=T1."Enabled" ("Disabled"), s=w416, f=T1."Disabled and Grayed Out" ("Disabled")) -> (s? t:f=w413:T1)
              n107 = Compound Arithmetic op=OR(w426, w425, w424, w423, w409) -> (w418:bool)
              n108 = Select(t=T1."Disabled and Grayed Out" ("Disabled"), s=w418, f=w413) -> (s? t:f=w412:T1)
              n109 = Bundle By Name(cluster=w437, "SSM"=w429, "Start SM Text"="START", "Star SM"=w434, "Pause SM"=w434, "Stop SM"=w434, "Abort SM"=w434, "Set SM"=w412) -> (w436:T4)
              n110 = Bundle By Name(cluster=w439, "P0"=w428, "P1"=w428, "P2"=w428, "P3"=w428, "P4"=w428, "P5"=w428, "P6"=w428, "P7"=w428, "P8"=w428, "P9"=w428, "P10"=w428, "P11"=w428, "P12"=w428, "P13"=w428, "P14"=w428, "P15"=w428, "Lambda Selector"=w429, "Calibrator Selector"=w429, "Set Waveplate"=w429, "Select Positions"=w428) -> (w438:T9)
            }
          }
        }
        frame True {
          w471 = T1."Disabled and Grayed Out" ("Disabled")
          # "Modo Síncrono"
          n111 = call-dynamic "Read Obs_state.vi"("error in (no error)"=w491, "S4ACS_GUI in"=w492) -> ("error out"=w477:errorcluster, "Obs_state"=w493:u32, "S4ACS_GUI out"=w461:refnum<class "S4GUI.lvclass">)  [unwired: 7 in]
          n112 = Equal?(x=w493, y=u32 0) -> (x = y?=w494:bool)
          n113 = case shown="True" w494 {
            tunnel: w493 -> [_ w550]
            tunnel: ["START" ("Caption.Text") "RESUME" ("Caption.Text")] -> w489
            tunnel: [w503 w552] -> w457
            tunnel: [w504 w552] -> w460
            tunnel: [w497 w552] -> w486
            tunnel: [w509 w551] -> w459
            tunnel: [w509 T1."Enabled" ("Disabled")] -> w485
            tunnel: [w509 w555] -> w484
            tunnel: [w501 w549] -> w483
            tunnel: [w498 w553] -> w464
            tunnel: [T1."Enabled" ("Disabled") T1."Disabled and Grayed Out" ("Disabled")] -> w467
            tunnel: w466 -> [w507 _]
            tunnel: [w506 w553] -> w465
            tunnel: [w499 w549] -> w463
            tunnel: [w499 w549] -> w462
            tunnel: [w497 w552] -> w455
            tunnel: w461 -> [w500 _]
            tunnel: w456 -> [w502 _]
            frame True {
              w499 = T1."Enabled" ("Disabled")
              w509 = T1."Disabled and Grayed Out" ("Disabled")
              # "Se estiver no modo \"ZERO\", desabilita \"Exptime\" de todos canais.\nSe estiver no modo \"TEST\", desabilita \"#Exp\" de todos e \"#Cycles\" do modo Síncrono."
              n114 = disable-structure shown="Enabled" {
                disable-tunnel: w500 -> [w520 w522]
                disable-tunnel: [w511 w532] -> w505
                frame Disabled {
                  n115 = Unbundle By Name(w520) -> ("AcquisitionA"=w519:refnum<class "Acquisition.lvclass">, "AcquisitionB"=w518:refnum<class "Acquisition.lvclass">, "AcquisitionC"=w517:refnum<class "Acquisition.lvclass">, "AcquisitionD"=w516:refnum<class "Acquisition.lvclass">)
                  n116 = call "Read connection.vi"("Server in"=w517) -> ("connection"=w513:bool)  [unwired: 8 in, 2 out]
                  n117 = call "Read connection.vi"("Server in"=w518) -> ("connection"=w514:bool)  [unwired: 8 in, 2 out]
                  n118 = call "Read connection.vi"("Server in"=w516) -> ("connection"=w512:bool)  [unwired: 8 in, 2 out]
                  n119 = call "Read connection.vi"("Server in"=w519) -> ("connection"=w515:bool)  [unwired: 8 in, 2 out]
                  n120 = Compound Arithmetic op=OR(w515, w514, w513, w512) -> (w511:bool)
                }
                frame Enabled {
                  n121 = Unbundle By Name(w522) -> ("AcquisitionA"=w527:refnum<class "Acquisition.lvclass">)
                  n122 = Unbundle By Name(w522) -> ("AcquisitionB"=w526:refnum<class "Acquisition.lvclass">)
                  n123 = Unbundle By Name(w522) -> ("AcquisitionC"=w525:refnum<class "Acquisition.lvclass">)
                  n124 = Unbundle By Name(w522) -> ("AcquisitionD"=w524:refnum<class "Acquisition.lvclass">)
                  n125 = Unbundle By Name(w522) -> ("Instrument.lvclass"=w523:refnum<class "Instrument.lvclass">)
                  n126 = call-dynamic "Read config running.vi"("Server in"=w527) -> ("config running"=w531:bool)  [unwired: 8 in, 2 out]
                  n127 = call-dynamic "Read config running.vi"("Server in"=w526) -> ("config running"=w530:bool)  [unwired: 8 in, 2 out]
                  n128 = call-dynamic "Read config running.vi"("Server in"=w525) -> ("config running"=w529:bool)  [unwired: 8 in, 2 out]
                  n129 = call-dynamic "Read config running.vi"("Server in"=w524) -> ("config running"=w528:bool)  [unwired: 8 in, 2 out]
                  n130 = call-dynamic "Read config running.vi"("Server in"=w523) -> ("config running"=w521:bool)  [unwired: 8 in, 2 out]
                  n131 = Compound Arithmetic op=OR(w531, w530, w529, w528, w521) -> (w532:bool)
                }
              }
              n132 = case shown="\"ZERO\"" w507 {
                tunnel: [T1."Disabled and Grayed Out" ("Disabled") T1."Enabled" ("Disabled") T1."Enabled" ("Disabled")] -> w506
                tunnel: [T1."Enabled" ("Disabled") T1."Disabled and Grayed Out" ("Disabled") T1."Enabled" ("Disabled")] -> w498
                tunnel: [T1."Enabled" ("Disabled") T1."Disabled and Grayed Out" ("Disabled") T1."Enabled" ("Disabled")] -> w496
                frame "ZERO" {
                }
                frame "TEST" {
                }
                frame Default {
                }
              }
              n133 = case shown="False" w505 {
                tunnel: [w533 w539] -> w504
                tunnel: [w536 w539] -> w503
                tunnel: w502 -> [w535 _]
                tunnel: [w534 w539] -> w501
                tunnel: [w534 w539] -> w497
                tunnel: w496 -> [w533 _]
                frame False {
                  w534 = T1."Enabled" ("Disabled")
                  n134 = case shown="True" w535 {
                    tunnel: [T1."Disabled and Grayed Out" ("Disabled") w538] -> w536
                    tunnel: w533 -> [_ w538]
                    frame False {
                      # "Photometric"
                    }
                    frame True {
                      # "Polarimetric, recebe enable\nda aba selecionada."
                    }
                  }
                }
                frame True {
                  w539 = T1."Disabled and Grayed Out" ("Disabled")
                }
              }
            }
            frame False {
              w553 = T1."Disabled and Grayed Out" ("Disabled")
              w552 = T1."Disabled and Grayed Out" ("Disabled")
              # "paused?"
              n135 = Equal?(x=w550, y=u32 400) -> (x = y?=w559:bool)
              n136 = case shown="True" w559 {
                tunnel: w552 -> [w562 w565]
                tunnel: [w562 T1."Enabled" ("Disabled")] -> w549
                tunnel: [T1."Enabled" ("Disabled") w565] -> w555
                tunnel: [T1."Enabled" ("Disabled") T1."Disabled and Grayed Out" ("Disabled")] -> w551
                frame False {
                }
                frame True {
                }
              }
            }
          }
          n137 = Bundle By Name(cluster=w490, "Start SM Text"=w489, "Star SM"=w483, "#Index Cycles"=T1."Enabled" ("Disabled"), "#Cycles"=w460, "Set SM"=w455, "SSM"=w455, "Pause SM"=w484, "Stop SM"=w459, "Abort SM"=w485) -> (w488:T4)
          n138 = Bundle By Name(cluster=w487, "P0"=w457, "P1"=w457, "P2"=w457, "P3"=w457, "P4"=w457, "P5"=w457, "P6"=w457, "P7"=w457, "P8"=w457, "P9"=w457, "P10"=w457, "P11"=w457, "P12"=w457, "P13"=w457, "P14"=w457, "P15"=w457, "Lambda Selector"=w486, "Calibrator Selector"=w486, "Set Waveplate"=w486, "Select Positions"=w457) -> (w478:T9)
          n139 = Bundle By Name(cluster=w482, "Exptime ch1"=w465, "Exp ch1"=w464, "#cycles ch1"=w471, "Start ch1 Text"="Sync", "Start ch1"=w471, "Pause ch1"=w471, "Stop ch1"=w471, "Abort ch1"=w471, "Set Cooler"=w463, "Set Temp"=w462) -> (w481:T5)
          n140 = Bundle By Name(cluster=w479, "Exptime ch2"=w465, "Exp ch2"=w464, "#cycles ch2"=w471, "Start ch2 Text"="Sync", "Start ch2"=w471, "Pause ch2"=w471, "Stop ch2"=w471, "Abort ch2"=w471, "Set Cooler"=w463, "Set Temp"=w462) -> (w480:T6)
          n141 = Bundle By Name(cluster=w473, "Exptime ch3"=w465, "Exp ch3"=w464, "#cycles ch3"=w471, "Start ch3 Text"="Sync" ("Start ch2 Text"), "Start ch3"=w471, "Pause ch3"=w471, "Stop ch3"=w471, "Abort ch3"=w471, "Set Cooler"=w463, "Set Temp"=w462) -> (w472:T7)
          n142 = Bundle By Name(cluster=w469, "Exptime ch4"=w465, "Exp ch4"=w464, "#cycles ch4"=w471, "Start ch4 Text"="Sync" ("Start ch2 Text"), "Start ch4"=w471, "Pause ch4"=w471, "Stop ch4"=w471, "Abort ch4"=w471, "Set Cooler"=w463, "Set Temp"=w462) -> (w468:T8)
        }
      }
      n143 = Bundle By Name(cluster=w7, "Cluster Mode Sync"=w36, "Cluster Mode CH1"=w35, "Cluster Mode CH2"=w34, "Cluster Mode CH3"=w28, "Cluster Mode CH4"=w27, "Cluster Polarimetry"=w29, "Cluster ExpMode.tab4"=w26) -> (w20:T2)
      n144 = Unbundle By Name(w6) -> ("mode Adm"=w19:bool)
      n145 = case shown="True" w19 {
        tunnel: [T1."Disabled and Grayed Out" ("Cluster AdmCCDSetup.param") T1."Enabled" ("Cluster AdmCCDSetup.param")] -> w18
        frame False {
        }
        frame True {
        }
      }
      n146 = Bundle By Name(cluster=w20, "Cluster AdmCCDsetup.param"=w18) -> (w10:T2)
      n147 = Bundle By Name(cluster=w6, "Cluster Disable"=w10) -> (w5:refnum<class "S4GUI.lvclass">)
    }
    frame Error {
    }
  }
  "error out" <- w3
  "S4ACS_GUI out" <- w1
